vi "Attempt to resolve locally.vi"(8 "error in (no error)":errorcluster, 11 "address":refnum<class "mDNS Hostname Network Address.lvclass">) -> (0 "error out":errorcluster, 3 "addresses out":refnum<class "Generic Network Address.lvclass">[](array[class]))   [LabVIEW 2020, in "NI_WFCN.lvlib" / "mDNS Hostname Network Address.lvclass"]
doc: "Use local facilities to resolve this address into the address which should be resolved next. For IP addresses, this typically does nothing. If a hostname is in /etc/hosts, this will look up its IP and return it. For DNS hostnames, this will return a DNS nameserver IP."
uses:
  <vilib>/net/WFCN/Addressing/mDNS Hostname Network Address/mDNS Hostname Network Address.lvclass
  e:/builds/penguin/labview/branches/2020/dev/dist/vi.lib/net/WFCN/Addressing/Generic Network Address/Generic Network Address.lvclass
  <vilib>/net/WFCN/Addressing/Generic Network Address/Generic Network Address.lvclass
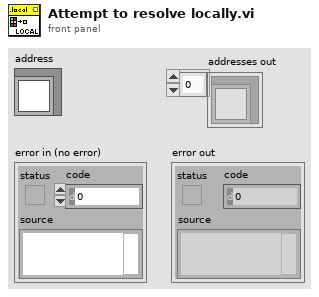
[diagram p1: front panel]
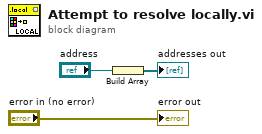
[diagram p0: block diagram]
diagram:
  n1 = Build Array("address") -> (→"addresses out":refnum<class "mDNS Hostname Network Address.lvclass">[])
  "error out" <- "error in (no error)"
